vi "Import Export - Export.vi"(8 "error in":errorcluster, 9 "Config Action":T1=enum."Cancel", 11 "Item Ref in":T2 format="%.0x") -> (0 "error out":errorcluster, 3 "Item Ref out":T2 format="%.0x")   [LabVIEW 2017, in "Scan Engine Custom Device.lvlib"]
uses:
  Scan Engine Custom Device.lvlib
  <vilib>/NI Veristand/Custom Device API/Custom Device Item Ref.ctl
  Type Defs/Host - Import Export Action.ctl
  <vilib>/NI/NI VeriStand Custom Device Import and Export Tool/ImportExport.lvlib
  <vilib>/NI Veristand/Custom Device API/Custom Device API.lvlib
panel:
  in  "Boolean":bool
  out "String":string
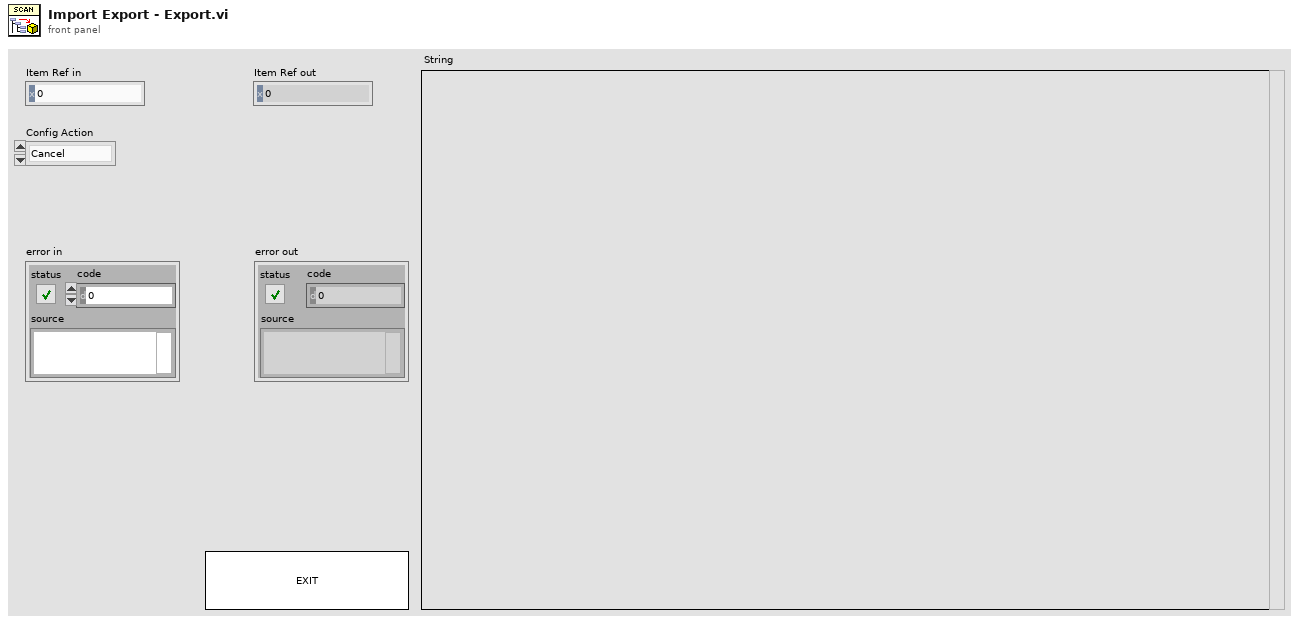
[diagram p1: front panel]
types:
  T1 = typedef "Scan Engine Custom Device.lvlib/Host - Import Export Action.ctl" = enum32{"Import", "Export", "Cancel"}
  T2 = typedef "Custom Device API.lvlib/Custom Device Item Ref.ctl" = u64
  T3 = enum32{"Invalid", "Standard", "Closed", "Hidden", "Minimized", "Maximized"}
  T4 = typedef "Advanced System Definition.lvlib/SysDef.Export.ctl" = cluster{"Version":string, "Tree":T5[]}
  T5 = typedef "Advanced System Definition.lvlib/TreeItem.ctl" = cluster{"Item Info":T6, "Parent Path":string[], "Properties":T11[]}
  T6 = typedef "Advanced System Definition.lvlib/TreeItem.Info.ctl" = cluster{"Name":string, "Description":string, "GUID":string, "Is Channel":bool, "Channel":T7, "Is Waveform":bool, "Waveform":T9}
  T7 = typedef "Custom Device API.lvlib/Custom Device Channel.ctl" = cluster{"Type":T8, "Units":string, "Default Value":dbl, "Faultable":bool, "Scalable":bool}
  T8 = typedef "Custom Device API.lvlib/Custom Device Channel Type.ctl" = enum16{"Input", "Output"}
  T9 = typedef "Custom Device API.lvlib/Custom Device Waveform.ctl" = cluster{"Data Type":T10, "Units":string}
  T10 = typedef "Custom Device API.lvlib/Custom Device Waveform DataType.ctl" = enum16{"Double", "Complex Double"}
  T11 = typedef "Advanced System Definition.lvlib/TreeItem.Property.ctl" = cluster{"Name":string, "Type":i32, "Value":variant}
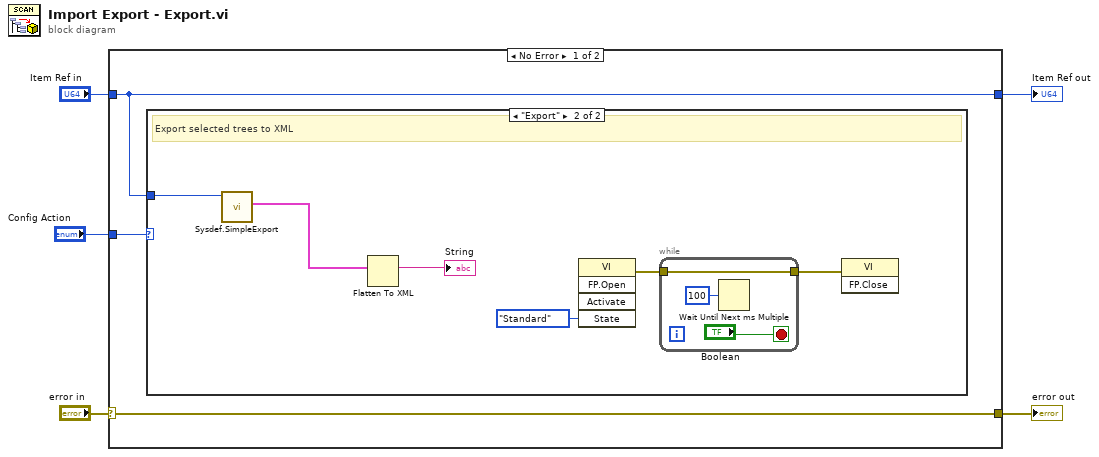
[diagram p0: block diagram]
diagram:
  n1 = case shown="No Error" "error in" {
    selector: "error in" -> [w8 w18]
    tunnel: [w8 w18] -> w4
    tunnel: [w6 w19] -> w3
    tunnel: "Item Ref in" -> [w6 w19]
    tunnel: "Config Action" -> [w7 _]
    frame No Error {
      n2 = case shown="\"Export\"" w7 {
        tunnel: w6 -> [_ w14]
        frame Default {
          # "Do nothing"
        }
        frame "Export" {
          # "Export selected trees to XML"
          n3 = call <vilib>:"Sysdef.SimpleExport.vi"("ID"=w14) -> ("Export"=w13:T4)  [unwired: 8 in, 2 out]
          n4 = Flatten To XML(anything=w13) -> (xml string=→"String":string)
          n5 = invoke class="VI" method="FP.Open"("State"=T3."Standard") -> (error out=w11:errorcluster)  [unwired: 4 in, 4 out]
          n6 = while {
            tunnel: [w15] -> w9
            tunnel: w11 -> [w15]
            stop <- "Boolean" stop-if-true
            n7 = Wait Until Next ms Multiple(millisecond multiple=u32 100) -> ()  [unwired: 1 out]
          }
          n8 = invoke class="VI" method="FP.Close"(error in=w9) -> ()  [unwired: 2 in, 3 out]
        }
      }
    }
    frame Error {
    }
  }
  "error out" <- w4
  "Item Ref out" <- w3
